vi "Handle Aliases Value Change.vi"(8 "error in (no error)":errorcluster, 9 "OldVal":T1[](array[typedef]), 10 "NewVal":T1[](array[typedef]), 11 "Aliases Ref in":T3 format="%.0x") -> (0 "error out":errorcluster, 1 "Duplicate Item":string, 2 "Duplicate Entry":bool, 3 "Aliases Ref out":T3 format="%.0x")   [LabVIEW 2020, in "Routing and Faulting System Explorer.lvlib"]
uses:
  Routing and Faulting System Explorer.lvlib
  <vilib>/NI VeriStand/Custom Device API/Custom Device Item Ref.ctl
  Alias.ctl
  Endpoint.ctl
  44871756-06de-413c-8c4c-f64fc17a87cb.vi
  <vilib>/NI VeriStand/Custom Device API/Custom Device API.lvlib
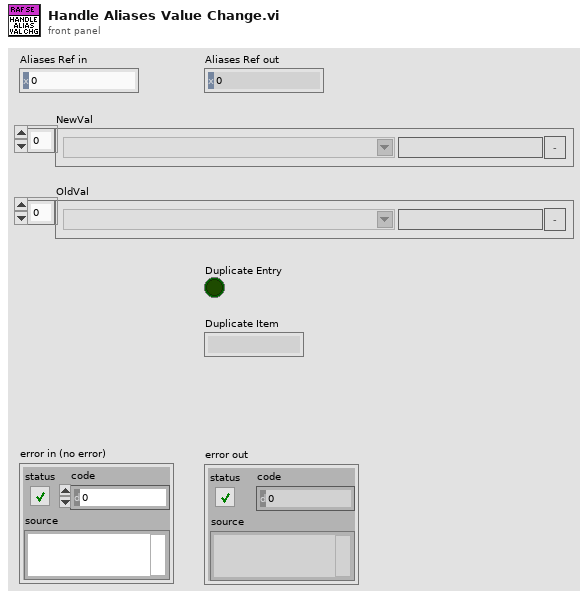
[diagram p1: front panel]
types:
  T1 = typedef "Routing and Faulting System Explorer.lvlib/Alias.ctl" = cluster{"Endpoint":T2, "Alias":string, "Remove":bool}
  T2 = typedef "Routing and Faulting System Explorer.lvlib/Endpoint.ctl" = string
  T3 = typedef "Custom Device API.lvlib/Custom Device Item Ref.ctl" = u64
  T4 = cluster{"Endpoint":bool, "Alias":bool, "Remove":bool}
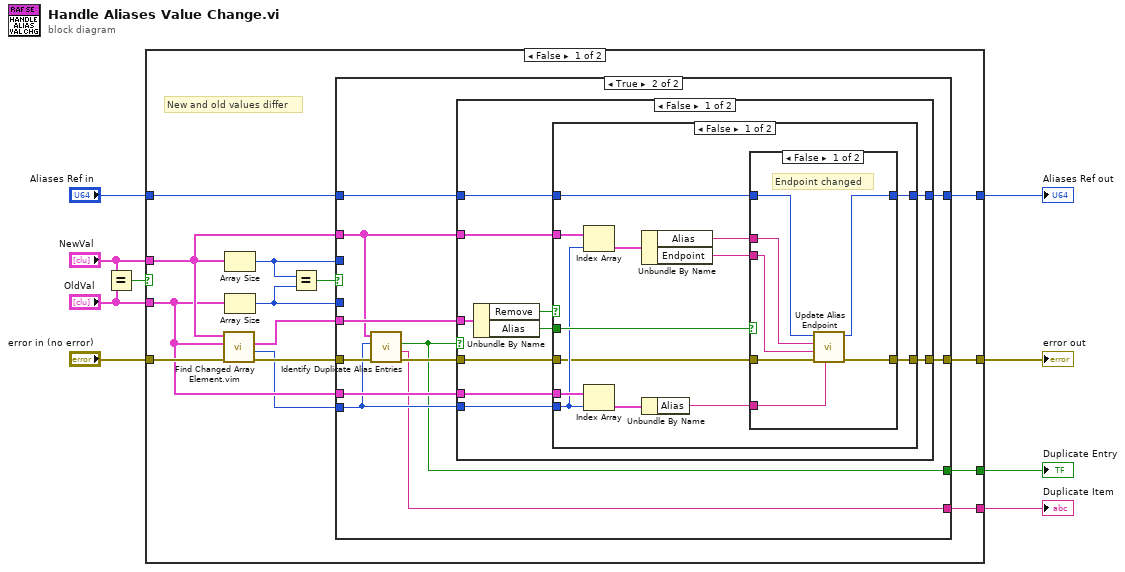
[diagram p0: block diagram]
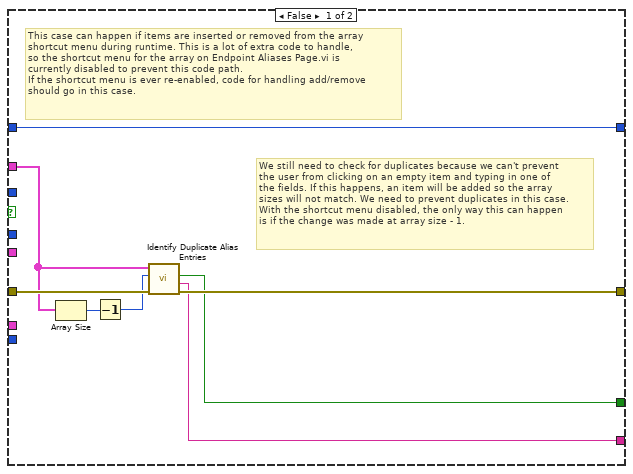
[diagram p2: hidden frame]
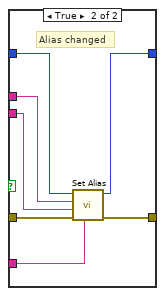
[diagram p3: hidden frame]
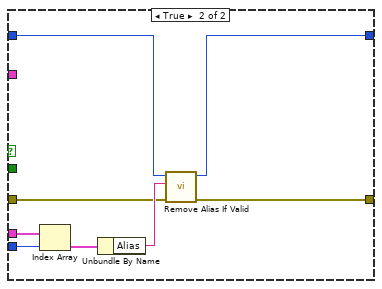
[diagram p4: hidden frame]
diagram:
  n1 = Equal?(x="NewVal", y="OldVal") -> (x = y?=w5:bool)
  n2 = case shown="False" w5 {
    tunnel: "error in (no error)" -> [w23 w90]
    tunnel: "Aliases Ref in" -> [w18 w91]
    tunnel: "NewVal" -> [w17 _]
    tunnel: "OldVal" -> [w16 _]
    tunnel: [w14 w90] -> w7
    tunnel: [w13 w91] -> w6
    tunnel: [w11 _] -> w2
    tunnel: [w10 _] -> w1
    frame False {
      # "New and old values differ"
      n3 = call "Find Changed Array Element.vim"("error in (no error)"=w23, "OldVal"=w16, "NewVal"=w17) -> ("error out"=w15:errorcluster, "Array Index"=w12:i32, "Element Changed"=w21:T4)  [unwired: 6 in]
      n4 = Array Size(array=w17) -> (size(s)=w20:i32)
      n5 = Array Size(array=w16) -> (size(s)=w19:i32)
      n6 = Equal?(x=w20, y=w19) -> (x = y?=w22:bool)
      n7 = case shown="True" w22 {
        tunnel: w12 -> [_ w34]
        tunnel: w21 -> [_ w42]
        tunnel: w20 -> [_ _]
        tunnel: w19 -> [_ _]
        tunnel: w18 -> [w31 w40]
        tunnel: w17 -> [w27 w35]
        tunnel: w16 -> [_ w41]
        tunnel: w15 -> [w30 w37]
        tunnel: [w29 w39] -> w14
        tunnel: [w31 w38] -> w13
        tunnel: [w25 w33] -> w11
        tunnel: [w24 w32] -> w10
        frame False {
          # "We still need to check for duplicates because we can't prevent\nthe user from clicking on an empty item and typing in one of\nthe fields. If this happens, an item will be added so the array\nsizes will not match. We need to prevent duplicates in this case.\nWith the shortcut menu disabled, the only way this can happen\nis if the change was made at array size - 1."
          # "This case can happen if items are inserted or removed from the array\nshortcut menu during runtime. This is a lot of extra code to handle,\nso the shortcut menu for the array on Endpoint Aliases Page.vi is\ncurrently disabled to prevent this code path.\nIf the shortcut menu is ever re-enabled, code for handling add/remove\nshould go in this case."
          n8 = Array Size(array=w27) -> (size(s)=w28:i32)
          n9 = Decrement(x=w28) -> (x-1=w26:i32)
          n10 = call "Identify Duplicate Alias Entries.vi"("error in (no error)"=w30, "Modified Index"=w26, "NewVal"=w27) -> ("error out"=w29:errorcluster, "Duplicate Message"=w24:string, "Duplicate Entry"=w25:bool)  [unwired: 6 in]
        }
        frame True {
          n11 = call "Identify Duplicate Alias Entries.vi"("error in (no error)"=w37, "Modified Index"=w34, "NewVal"=w35) -> ("error out"=w36:errorcluster, "Duplicate Message"=w32:string, "Duplicate Entry"=w33:bool)  [unwired: 6 in]
          n12 = case shown="False" w33 {
            tunnel: w42 -> [w52 _]
            tunnel: w41 -> [w50 _]
            tunnel: w40 -> [w49 w88]
            tunnel: [w47 w89] -> w39
            tunnel: [w46 w88] -> w38
            tunnel: w36 -> [w45 w89]
            tunnel: w35 -> [w44 _]
            tunnel: w34 -> [w43 _]
            frame False {
              n13 = Unbundle By Name(w52) -> ("Remove"=w51:bool, "Alias"=w48:bool)
              n14 = case shown="False" w51 {
                tunnel: w43 -> [w59 w86]
                tunnel: w49 -> [w56 w83]
                tunnel: w50 -> [w60 w87]
                tunnel: w48 -> [w61 _]
                tunnel: w44 -> [w65 _]
                tunnel: w45 -> [w55 w82]
                tunnel: [w54 w81] -> w47
                tunnel: [w53 w80] -> w46
                frame False {
                  n15 = Index Array(array=w65, index=w59) -> (element=w64:T1)
                  n16 = Index Array(array=w60, index=w59) -> (element=w58:T1)
                  n17 = Unbundle By Name(w64) -> ("Alias"=w63:string, "Endpoint"=w62:T2)
                  n18 = Unbundle By Name(w58) -> ("Alias"=w57:string)
                  n19 = case shown="False" w61 {
                    tunnel: w63 -> [w70 w77]
                    tunnel: w62 -> [w69 w76]
                    tunnel: w57 -> [w66 w74]
                    tunnel: w56 -> [w71 w78]
                    tunnel: w55 -> [w72 w79]
                    tunnel: [w68 w75] -> w54
                    tunnel: [w67 w73] -> w53
                    frame False {
                      # "Endpoint changed"
                      n20 = call "Update Alias Endpoint.vi"("Previous Alias"=w66, "error in (no error)"=w72, "Endpoint"=w69, "Alias"=w70, "Aliases Ref in"=w71) -> ("error out"=w68:errorcluster, "Aliases Ref out"=w67:T3)  [unwired: 5 in]
                    }
                    frame True {
                      # "Alias changed"
                      n21 = call "Set Alias.vi"("Previous Alias"=w74, "error in (no error)"=w79, "Endpoint"=w76, "Alias"=w77, "Aliases Ref in"=w78) -> ("error out"=w75:errorcluster, "Aliases Ref out"=w73:T3)  [unwired: 5 in]
                    }
                  }
                }
                frame True {
                  n22 = Index Array(array=w87, index=w86) -> (element=w85:T1)
                  n23 = Unbundle By Name(w85) -> ("Alias"=w84:string)
                  n24 = call "Remove Alias If Valid.vi"("error in (no error)"=w82, "Alias"=w84, "Aliases Ref in"=w83) -> ("error out"=w81:errorcluster, "Aliases Ref out"=w80:T3)  [unwired: 7 in]
                }
              }
            }
            frame True {
              # "Either endpoint or alias is duplicated. Do nothing, but report duplicates"
            }
          }
        }
      }
    }
    frame True {
      # "New and old values are the same. Do nothing"
    }
  }
  "Aliases Ref out" <- w6
  "error out" <- w7
  "Duplicate Entry" <- w2
  "Duplicate Item" <- w1
